vi "MoveAbsMultiple.vi"(0 "controller in":refnum<k24>, 5 "axis names":string[](array[string]), 7 "speeds":dbl[](array[numeric]), 9 "distances":dbl[](array[numeric]), 11 "error in (no error)":errorcluster, 12 "return immediately":bool) -> (4 "controller out":refnum<k24>, 15 "error out":errorcluster)   [LabVIEW 2010]
uses:
  c:/aerotech/controller/5.xx.xxx/ensemble/pc/labview/2010/bin/Aerotech.Ensemble.dll
  bin/Aerotech.Ensemble.dll
  c:/aerotech/controller/5.xx.xxx/ensemble/pc/labview/2010/bin/Aerotech.Ensemble.LabVIEW.dll
  bin/Aerotech.Ensemble.LabVIEW.dll
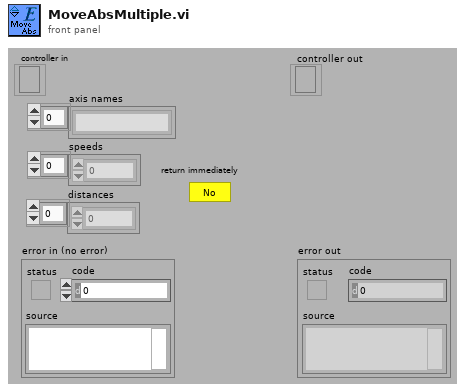
[diagram p1: front panel]
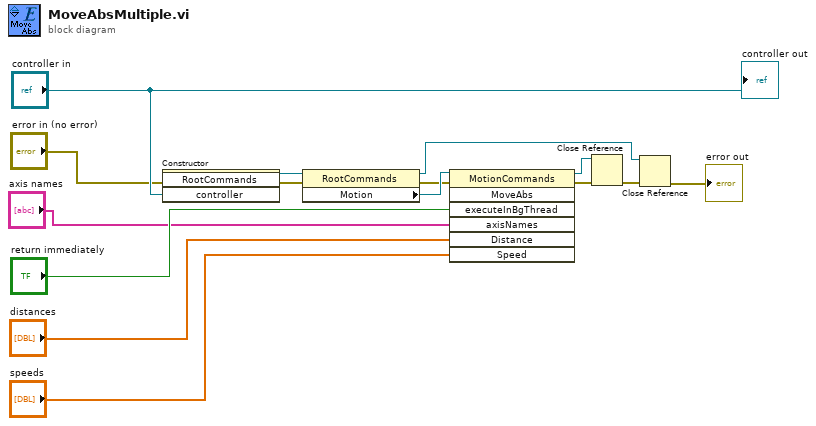
[diagram p0: block diagram]
diagram:
  n1 = constructor class="RootCommands"(error in="error in (no error)", "controller"="controller in") -> (reference out=w9:refnum<k24>, error out=w8:errorcluster)  [unwired: 2 in, 2 out]
  n2 = property class="RootCommands"(reference=w9, error in=w8) -> (reference out=w4:refnum<k24>, error out=w10:errorcluster, "Motion"=w11:refnum<k24>)
  n3 = invoke class="MotionCommands" method="MoveAbs"(reference=w11, error in=w10, "executeInBgThread"="return immediately", "axisNames"="axis names", "Distance"="distances", "Speed"="speeds") -> (reference out=w6:refnum<k24>, error out=w7:errorcluster)  [unwired: 1 in, 5 out]
  n4 = Close Reference(reference=w6, error in (no error)=w7) -> (error out=w5:errorcluster)
  n5 = Close Reference(reference=w4, error in (no error)=w5) -> (error out=→"error out":errorcluster)
  "controller out" <- "controller in"
